vi "Edit Time Entry.vi"() -> ()   [LabVIEW 2020, in "Main_Process.lvlib"]
uses:
  Main_Process.lvlib
panel:
  in  "End Time":timestamp format="%<%x %.3X>T"
  in  "Start Time":timestamp format="%<%x %.3X>T"
  in  "Comment":string
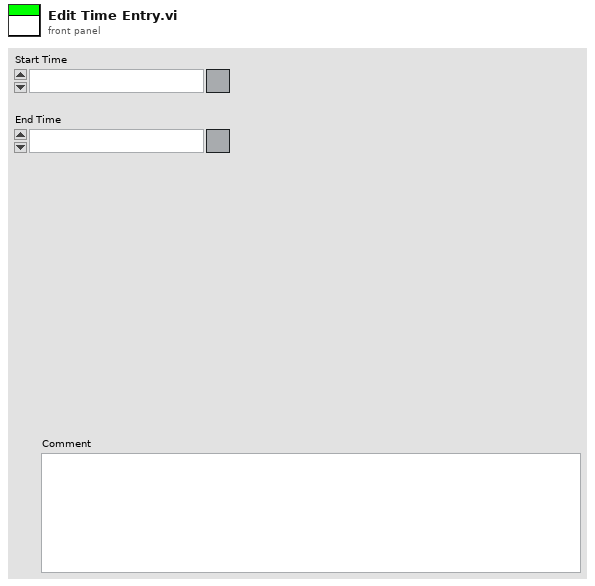
[diagram p1: front panel]
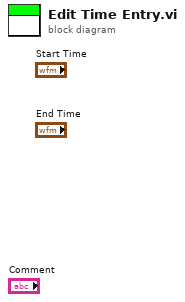
[diagram p0: block diagram]
diagram:
